vi "Actor Core.vi"(8 "error in":errorcluster, 11 "CameraTestingUI in":refnum<class "CameraTestingUI.lvclass">) -> (0 "error out":errorcluster, 3 "Actor out":refnum<class "Actor.lvclass">)   [LabVIEW 2020, in "CameraTestingUI.lvlib" / "CameraTestingUI.lvclass"]
doc: "(<B>Filename</B>: Actor Framework.lvlib:Actor.lvclass:Actor Core.vi)\n\nReceives messages to the actor, reacts to them, and initiates any error handling that may shut the actor down.\n\nDescendant classes may override this VI to append parallel tasks for the actor to complete while it handles messages. Overrides use the Call Parent Class Method node."
uses:
  CameraTestingUI.lvclass
  <vilib>/ActorFramework/Actor/Actor.lvclass
  Private/TypeDef/ConnectCamera.ctl
  Private/TypeDef/DisconnectCamera.ctl
  Private/TypeDef/CommandParameters.ctl
  Private/TypeDef/SetParams.ctl
  Private/TypeDef/GetParams.ctl
  CameraTestingUI.lvclass/CameraTestingUI.ctl
panel:
  out "Quit":T1
  out "StoptRec":T2
  out "StartRec":T2
  out "Snap":T1
  out "ValueRead":string caption="Value Read"
  in  "CommandParameters":T3
  in  "GetParameter":T4
  in  "SetParameter":T5
  out "DisconnectCamera":T2
  out "ConnectCamera":T1
  out "StatusLog":string caption="Status Log"
  # "Parameters"
  # "Actions"
  # "New value : set to"
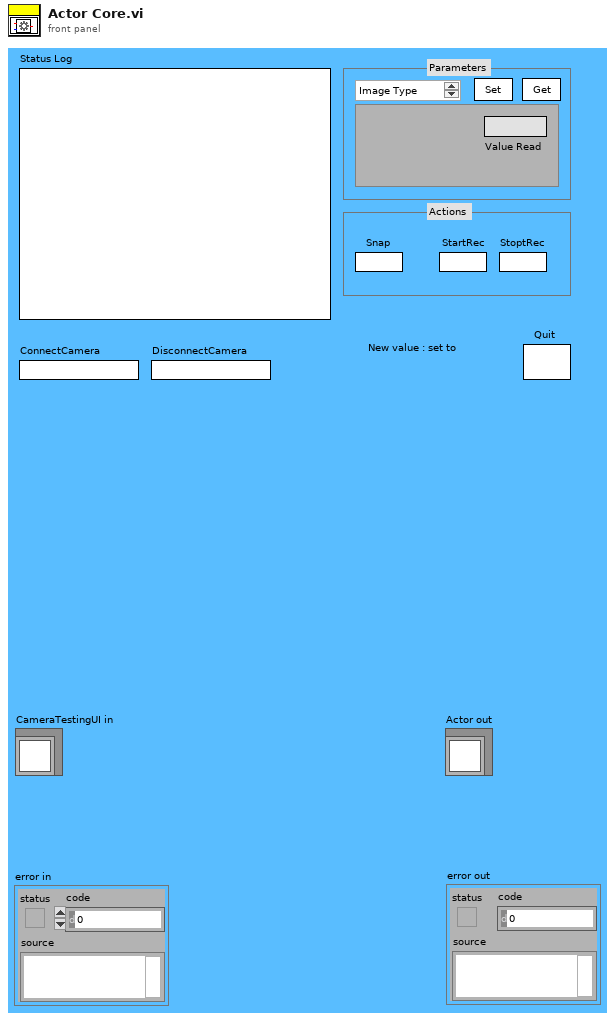
[diagram p1: front panel]
types:
  T1 = typedef "CameraTestingUI.lvlib/CameraTestingUI.lvclass/ConnectCamera.ctl" = bool
  T2 = typedef "CameraTestingUI.lvlib/CameraTestingUI.lvclass/DisconnectCamera.ctl" = bool
  T3 = typedef "CameraTestingUI.lvlib/CameraTestingUI.lvclass/CommandParameters.ctl" = enum32{"Image Type", "Resolution", "Frame Rate"}
  T4 = typedef "CameraTestingUI.lvlib/CameraTestingUI.lvclass/GetParams.ctl" = bool
  T5 = typedef "CameraTestingUI.lvlib/CameraTestingUI.lvclass/SetParams.ctl" = bool
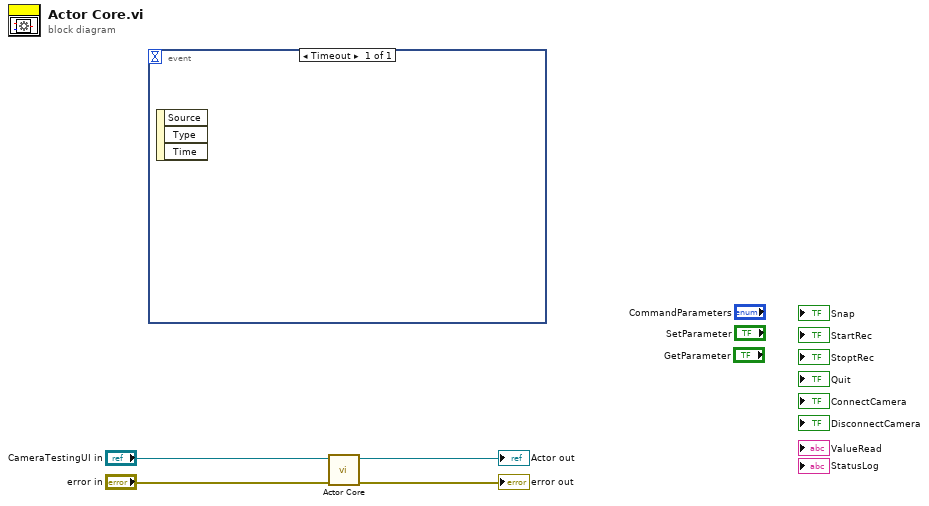
[diagram p0: block diagram]
diagram:
  n1 = event shown="[0] Timeout" {
    selector: _ -> [_]
    dyn-events: _ -> [_]
    timeout: _ -> [_]
    event Timeout {
      n2 = event-data() -> ()  [unwired: 1 in, 3 out]
    }
  }
  n3 = call-parent "Actor Core.vi"("error in"="error in", "Actor in"="CameraTestingUI in") -> ("error out"=→"error out":errorcluster, "Actor out"=→"Actor out":refnum<class "Actor.lvclass">)  [unwired: 8 in]
